vi "Ver 1.1.vi"() -> ()   [LabVIEW 2015]
uses:
  Program Files (x86)/National Instruments/LabVIEW 2016/instr.lib/Keithley 2000/Keithley 2000.lvlib
  Program Files (x86)/National Instruments/LabVIEW 2016/instr.lib/Keithley622xLV2009_0/Keithley 622x LV 2009/Keithley 622x.lvlib
  Program Files (x86)/National Instruments/LabVIEW 2016/instr.lib/Keithley622xLV2009_0/Keithley 622x LV 2009/Utility/Typedefs/KE622x -- Instrument Type.ctl
  Program Files (x86)/National Instruments/LabVIEW 2016/instr.lib/Keithley622xLV2009_0/Keithley 622x LV 2009/Configure/Source/Typedefs/KE622x -- Current Level.ctl
  Program Files (x86)/National Instruments/LabVIEW 2016/instr.lib/Keithley622xLV2009_0/Keithley 622x LV 2009/Configure/Source/Typedefs/KE622x -- Voltage Limit.ctl
  Program Files (x86)/National Instruments/LabVIEW 2016/instr.lib/Keithley 2000/Public/Configure/Configure DC Volts.vi
  Program Files (x86)/National Instruments/LabVIEW 2016/instr.lib/Keithley622xLV2009_0/Keithley 622x LV 2009/Typedefs/KE622x -- On Off Control.ctl
  Program Files (x86)/National Instruments/LabVIEW 2016/instr.lib/Keithley622xLV2009_0/Keithley 622x LV 2009/Configure/Source/Typedefs/KE622x -- Current Range.ctl
  Program Files (x86)/National Instruments/LabVIEW 2016/instr.lib/Keithley622xLV2009_0/Keithley 622x LV 2009/Configure/Source/Typedefs/KE622x -- Current Ranges.ctl
panel:
  out "Error Code":string
  in  "File name":string
  in  "Comments":string
  in  "Root Path":path=path "C:/"
  out "file":refnum<file>
  in  "Custom Range (0 V) 2":dbl format="%#_6p"
  in  "Auto\nRange 2":bool
  out "2000":refnum<visa-resource-name>
  out "6221":refnum<visa-resource-name>
  in  "Floating-point file recording":bool
  in  "Step  (A)":dbl=5e-05 format="%#_3p"
  in  "Stop\ncurrent (A)":dbl=0.002 format="%#_6p"
  in  "Start \ncurrent (A)":dbl=0.001 format="%#_6p"
  out "?":string
  out "?":string
  in  "Change Volt Ampers":bool
  in  "Check For SCPI Errors? (T)":bool=TRUE
  out "Interlock Tripped?":bool
  out "Compliance?":bool
  in  "Turn Off Output \nIf Compliance?":bool=TRUE
  in  "Turning ON/OFF\ncurrent output":T1=enum."On"
  out "?":cluster{dbl[], dbl[]}[](graph)
  in  "Range Selection":T2={"Auto Range?"=TRUE, "Man / Selected\nRange"=enum."2nA"}
  in  "Voltage Limit (V) 3":T4=10.0 min=0.1 max=105.0 step=0.01 format="%.2p"
  in  "Interval (s)":dbl=1.0 min=1.0
  out "?":cluster{T4[], T4[]}(graph)
  # "FILE CONFIGURATION"
  # "START, STOP, STEP, CONFIGURATION"
  # "KEITHLEY 6221 CONFIGURATION (ADMIN ONLY)"
  # "IF ON"
  # "I don't know what the hell it is,\njust don't touch it"
  # "Compliance = Limiting output voltage\nThis switch determines if we want to switch \noff the current output if wee exceed compliance"
  # "There is a safe switch at \nthe back of the instrument \nThis indicator shows if it is on"
  # "You have hit a damn jackpot \nby exceeding the limited voltage\nCongrats"
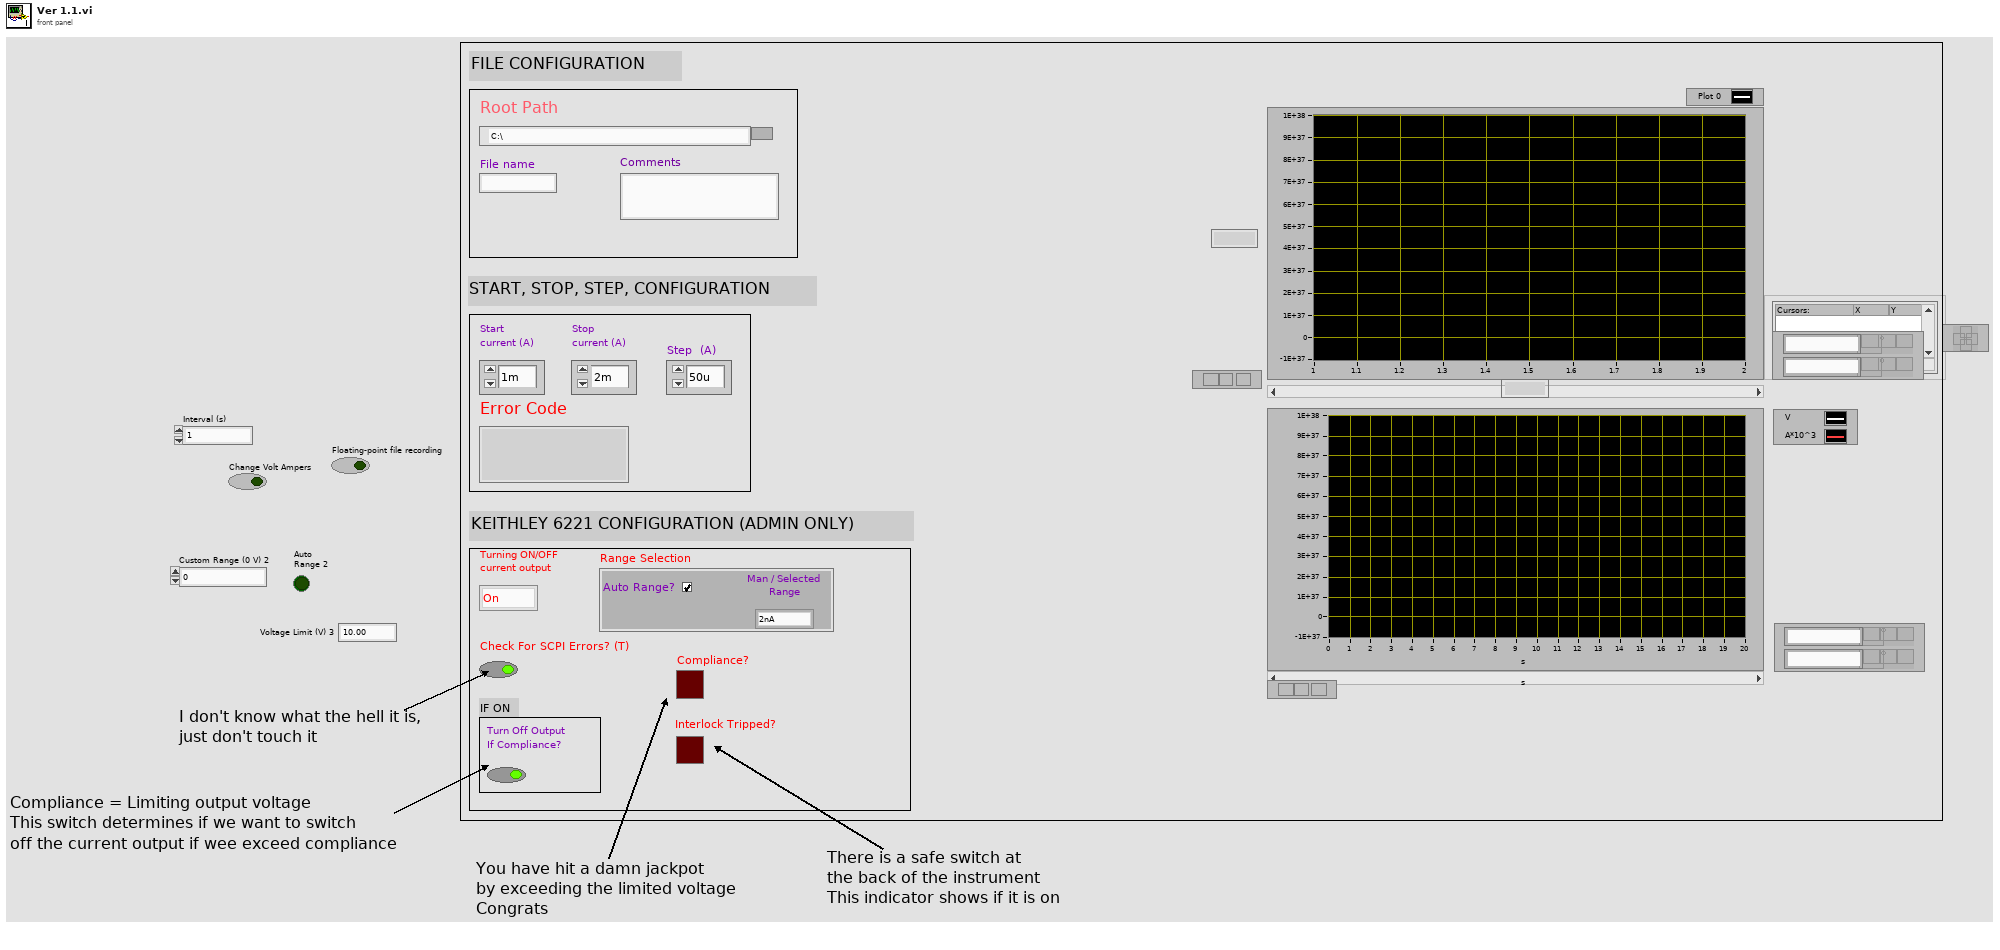
[diagram p1: front panel]
types:
  T1 = typedef "Keithley 622x.lvlib/KE622x -- On Off Control.ctl" = enum16{"Off", "On"}
  T2 = typedef "Keithley 622x.lvlib/KE622x -- Current Range.ctl" = cluster{"Auto Range?":bool, "Man / Selected\nRange":T3}
  T3 = typedef "Keithley 622x.lvlib/KE622x -- Current Ranges.ctl" = enum16{"2nA", "20nA", "200nA", "2uA", "20uA", "200uA", "2mA", "20mA", "100mA"}
  T4 = typedef "Keithley 622x.lvlib/KE622x -- Voltage Limit.ctl" = dbl
  T5 = enum16{"open", "replace", "create", "open or create", "replace or create", "replace or create with confirmation"}
  T6 = typedef "Keithley 622x.lvlib/KE622x -- Instrument Type.ctl" = enum16{"KE6220", "KE6221"}
  T7 = typedef "Keithley 622x.lvlib/KE622x -- Current Level.ctl" = dbl
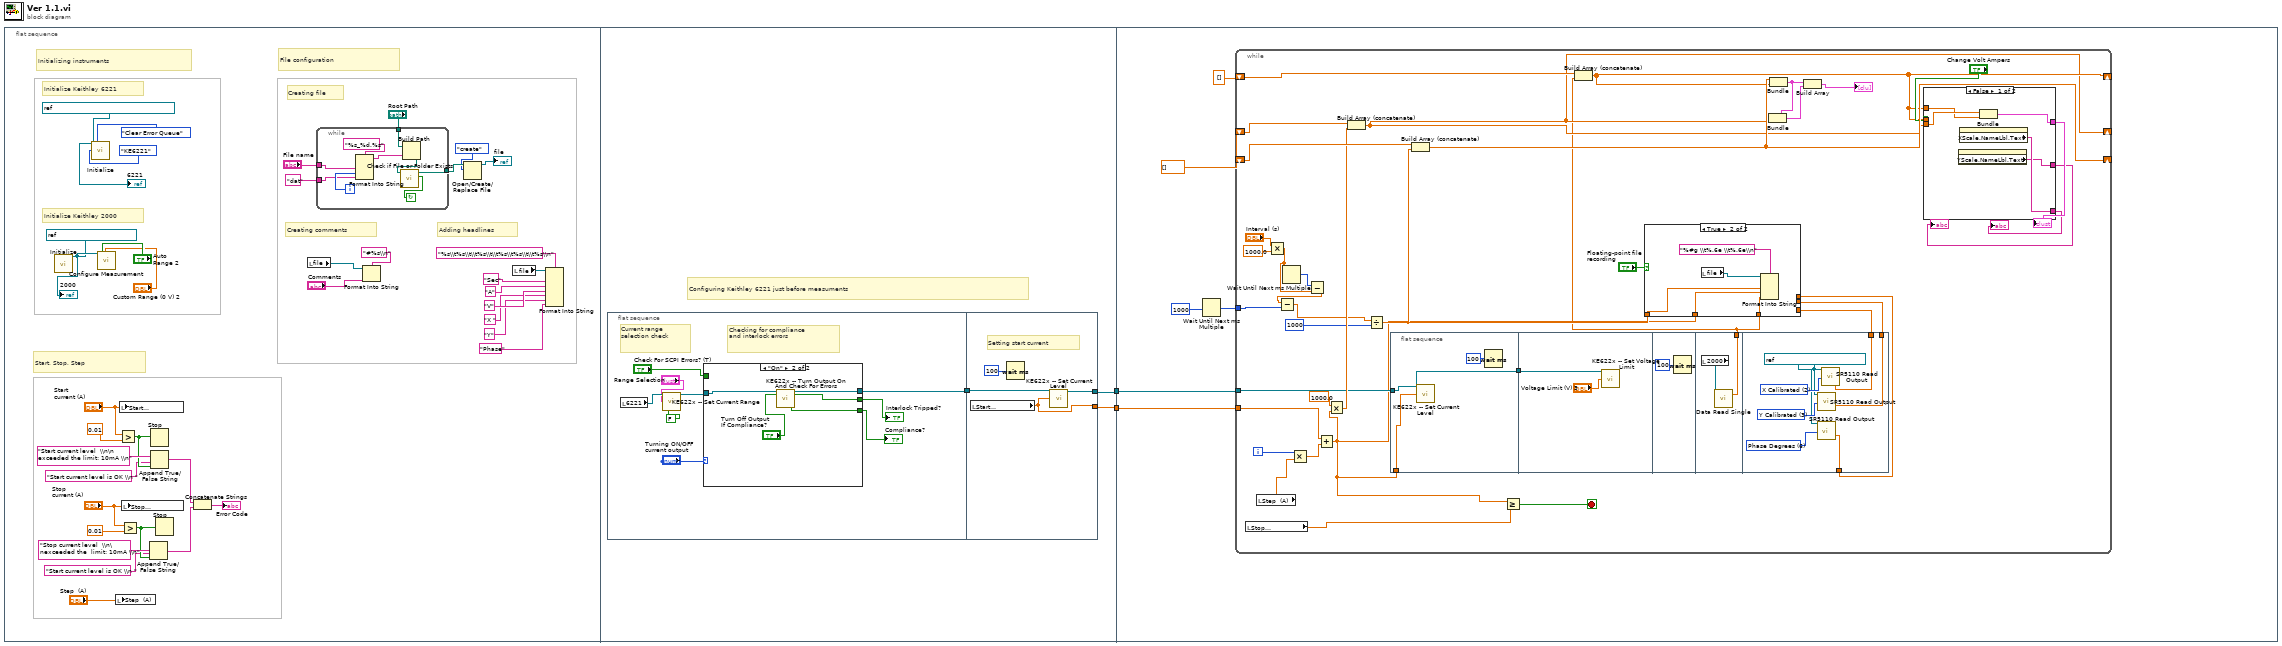
[diagram p0: block diagram]
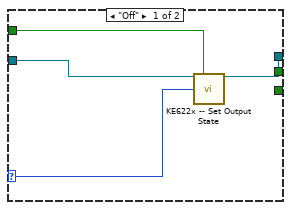
[diagram p2: hidden frame]
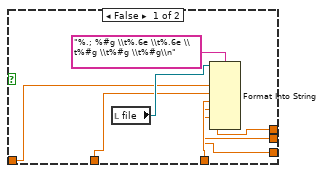
[diagram p3: hidden frame]
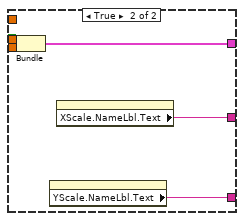
[diagram p4: hidden frame]
diagram:
  n1 = flat-sequence {
    tunnel: [w53] -> w2
    tunnel: [w52] -> w1
    tunnel: w2 -> [w76]
    tunnel: w1 -> [w77]
    frame #0 {
      # "Start, Stop, Step"
      # "Adding headlines"
      # "Creating file"
      # "Initializing instruments"
      # "Creating comments"
      # "File configuration"
      # "Initialize Keithley 2000"
      # "Initialize Keithley 6221"
      n2 = call "Initialize.vi"("VISA resource name"=refnum<visa-resource-name> "KEITHLEY_MULTIMETER") -> ("VISA resource name out"=w37:refnum<visa-resource-name>)  [unwired: 17 in, 1 out]
      "2000" <- w37
      n3 = call "Initialize.vi"("VISA resource name"=refnum<visa-resource-name> "KEITHLEY_DC_AC_CURRENT_SOURCE", "Error Queue Option"=enum16{"Clear Error Queue", "Error Query"}."Clear Error Queue", "Instrument Type"=KE622x_--_Instrument_Type."KE6221") -> ("VISA resource name out"=→"6221":refnum<visa-resource-name>)  [unwired: 11 in, 1 out]
      n4 = call-poly "Configure Measurement.vi"("VISA resource name"=w37, "Auto Range? (T: Auto)"="Auto\nRange 2", "Custom Range (0 V)"="Custom Range (0 V) 2") -> ()  [unwired: 15 in, 2 out]
      n5 = local write "Step  (A)"("Step  (A)") -> ()
      n6 = local write "Start \ncurrent (A)"("Start \ncurrent (A)") -> ()
      n7 = Greater?(x="Start \ncurrent (A)", y=T4 0.01) -> (0:w10:bool)
      n8 = Greater?(x="Stop\ncurrent (A)", y=T4 0.01) -> (0:w8:bool)
      n9 = local write "Stop\ncurrent (A)"("Stop\ncurrent (A)") -> ()
      n10 = Append True/False String(1:w8, 2:"Start current level is OK \\n " ("false string"), 3:"Stop current level  \\n\nexceeded the  limit: 10mA \\n" ("String")) -> (0:w4:string)  [unwired: 1 in]
      n11 = Stop(stop? (T)=w10) -> ()
      n12 = Append True/False String(1:w10, 2:"Start current level is OK \\n " ("false string"), 3:"Start current level  \\n\n exceeded the limit: 10mA \\n" ("String")) -> (0:w5:string)  [unwired: 1 in]
      n13 = Stop(stop? (T)=w8) -> ()
      n14 = Concatenate Strings(w5, w4) -> (→"Error Code":string)
      n15 = local read "file"() -> (w21:refnum<file>)
      n16 = while {
        tunnel: "dat" ("format string") -> [w48]
        tunnel: "File name" -> [w47]
        tunnel: "Root Path" -> [w45]
        tunnel: [w43] -> w31
        i -> [w49]
        stop <- w42 continue-if-true
        n17 = Format Into String(format string="%s_%d.%s", w47, w49, w48) -> (resulting string=w46:string)  [unwired: 2 in, 1 out]
        n18 = Build Path(base path=w45, name or relative path=w46) -> (appended path=w44:path)
        n19 = call <vilib>:"Check if File or Folder Exists.vi"("path"=w44) -> ("file or folder exists?"=w42:bool, "dup path"=w43:path)  [unwired: 8 in, 1 out]
      }
      n20 = Format Into String(format string="#%s\\n", initial string=w21, "Comments") -> ()  [unwired: 1 in, 2 out]
      n21 = Open/Create/Replace File(file path (use dialog)=w31, operation (0:open)=T5."create") -> (refnum out=→"file":refnum<file>)  [unwired: 4 in, 2 out]
      n22 = local read "file"() -> (w18:refnum<file>)
      n23 = Format Into String(format string="%s\\t%s\\t\\t%s\\t\\t%s\\t%s\\t\\t%s\\n", initial string=w18, "Sec" ("input 1"), "A" ("input 2"), "V" ("input 3"), "X " ("input 3"), "Y" ("input 3"), "Phase" ("input 3")) -> ()  [unwired: 1 in, 2 out]
    }
    frame #1 {
      # "Configuring Keithley 6221 just before measuments"
      n24 = flat-sequence {
        tunnel: [w54] -> w51
        tunnel: [w72] -> w53
        tunnel: [w74] -> w52
        tunnel: w51 -> [w73]
        frame #0 {
          # "Current range \nselection check"
          # "Checking for compliance\nand interlock errors"
          n25 = local read "6221"() -> (w57:refnum<visa-resource-name>)
          n26 = call "KE622x -- Set Current Range.vi"("Resource In"=w57, "Current Range In"="Range Selection", "Read Back Set Values? (T)"=FALSE) -> ("Resource Out (dupl)"=w62:refnum<visa-resource-name>)  [unwired: 10 in, 2 out]
          n27 = case shown="\"On\"" "Turning ON/OFF\ncurrent output" {
            selector: "Turning ON/OFF\ncurrent output" -> [w66 _]
            tunnel: [_ w70] -> w60
            tunnel: [_ w69] -> w61
            tunnel: "Check For SCPI Errors? (T)" -> [w65 _]
            tunnel: w62 -> [w63 w68]
            tunnel: [w64 w67] -> w54
            frame "Off" {
              n28 = call "KE622x -- Set Output State.vi"("Resource In"=w63, "Check For SCPI Errors? (T)"=w65, "Output State"=w66) -> ("Resource Out (dupl)"=w64:refnum<visa-resource-name>)  [unwired: 11 in, 1 out]
            }
            frame "On" {
              n29 = call "KE622x -- Turn Output On And Check For Errors.vi"("Resource In"=w68, "Turn Off Output If Compliance?"="Turn Off Output \nIf Compliance?") -> ("Resource Out (dupl)"=w67:refnum<visa-resource-name>, "Interlock Tripped?"=w70:bool, "Compliance?"=w69:bool)  [unwired: 10 in, 1 out]
            }
          }
          "Interlock Tripped?" <- w60
          "Compliance?" <- w61
        }
        frame #1 {
          # "Setting start current"
          n30 = local read "Start \ncurrent (A)"() -> (w72:dbl)
          n31 = Wait (ms)(milliseconds to wait=u32 100) -> ()  [unwired: 1 out]
          n32 = call "KE622x -- Set Current Level.vi"("Resource In"=w73, "Current Level (A) In"=w72) -> ("Resource Out (dupl)"=w74:refnum<visa-resource-name>)  [unwired: 11 in, 2 out]
        }
      }
    }
    frame #2 {
      n33 = Wait Until Next ms Multiple(millisecond multiple=u32 1000) -> (millisecond timer value=w78:u32)
      n34 = while {
        shift-right: [w110] -> _
        shift-left: dbl[] [] -> [w119]
        shift-right: [w115] -> _
        shift-left: _ -> [w117]
        shift-right: [w105] -> _
        shift-left: T7[] [] -> [w116]
        tunnel: w77 -> [w98]
        tunnel: w78 -> [w93]
        tunnel: w76 -> [w84]
        i -> [w107]
        stop <- w82 stop-if-true
        n35 = local read "Stop\ncurrent (A)"() -> (w83:dbl)
        n36 = local read "Step  (A)"() -> (w85:dbl)
        n37 = Multiply(x="Interval (s)", y=1000.0) -> (x*y=w94:dbl)
        n38 = Wait Until Next ms Multiple(millisecond multiple=w94) -> (millisecond timer value=w97:u32)
        n39 = Multiply(x=w107, y=w85) -> (x*y=w106:dbl)
        n40 = Subtract(x=w97, y=w94) -> (x-y=w92:dbl)
        n41 = Subtract(x=w92, y=w93) -> (x-y=w91:dbl)
        n42 = Add(x=w84, y=w106) -> (x+y=w95:dbl)
        n43 = Multiply(x=T4 1000.0, y=w95) -> (x*y=w104:T4)
        n44 = Build Array (concatenate)(w116, w104) -> (w105:T4[])
        n45 = Divide(x=w91, y=1000) -> (x/y=w101:dbl)
        n46 = flat-sequence {
          tunnel: w95 -> [w136]
          tunnel: w98 -> [w135]
          tunnel: [w134] -> w96
          tunnel: w96 -> [w137]
          tunnel: [w140] -> w88
          tunnel: [w148] -> w89
          tunnel: [w143] -> w87
          tunnel: [w142] -> w86
          frame #0 {
            n47 = call "KE622x -- Set Current Level.vi"("Resource In"=w135, "Current Level (A) In"=w136) -> ("Resource Out (dupl)"=w134:refnum<visa-resource-name>)  [unwired: 11 in, 2 out]
            n48 = Wait (ms)(milliseconds to wait=u32 100) -> ()  [unwired: 1 out]
          }
          frame #1 {
            n49 = call "KE622x -- Set Voltage Limit.vi"("Resource In"=w137, "Voltage Limit (V)"="Voltage Limit (V) 3") -> ()  [unwired: 12 in, 2 out]
          }
          frame #2 {
            n50 = Wait (ms)(milliseconds to wait=u32 100) -> ()  [unwired: 1 out]
          }
          frame #3 {
            n51 = local read "2000"() -> (w141:refnum<visa-resource-name>)
            n52 = call "Data Read Single.vi"("VISA resource name"=w141) -> ("Measurement"=w140:dbl)  [unwired: 14 in, 4 out]
          }
          frame #4 {
            w145 = u16 6 items=["X %", "Y %", "X Calibrated", "Y Calibrated", "Mag %", "Mag Calibrated", "Phase Degrees", "Ratio", "ADC 1", "ADC 2", "ADC 3", "ADC 4 ", "Noise %", "Noise Calibrated", "Ref Frequency", "", ""] ("Display Type")
            w146 = u16 3 items=["X %", "Y %", "X Calibrated", "Y Calibrated", "Mag %", "Mag Calibrated", "Phase Degrees", "Ratio", "ADC 1", "ADC 2", "ADC 3", "ADC 4 ", "Noise %", "Noise Calibrated", "Ref Frequency", "", ""] ("Display Type")
            w147 = u16 2 items=["X %", "Y %", "X Calibrated", "Y Calibrated", "Mag %", "Mag Calibrated", "Phase Degrees", "Ratio", "ADC 1", "ADC 2", "ADC 3", "ADC 4 ", "Noise %", "Noise Calibrated", "Ref Frequency", "", ""] ("Display Type")
            w144 = refnum<visa-resource-name> "LOCK_IN_5110_PRINCETON" ("VISA session (for class)")
            n53 = call "SR5110 Read Output"("VISA session (for class)"=w144, "Display Type"=w145) -> ("Output (FP)"=w142:dbl)  [unwired: 9 in, 8 out]
            n54 = call "SR5110 Read Output"("VISA session (for class)"=w144, "Display Type"=w146) -> ("Output (FP)"=w143:dbl)  [unwired: 9 in, 8 out]
            n55 = call "SR5110 Read Output"("VISA session (for class)"=w144, "Display Type"=w147) -> ("Display"=w148:dbl)  [unwired: 9 in, 8 out]
          }
        }
        n56 = Build Array (concatenate)(w117, w101) -> (w115:dbl[])
        n57 = Greater Or Equal?(x=w95, y=w83) -> (x >= y?=w82:bool)
        n58 = Build Array (concatenate)(w119, w88) -> (w110:dbl[])
        n59 = case shown="True" "Floating-point file recording" {
          tunnel: w101 -> [w123 w130]
          tunnel: w88 -> [w125 w129]
          tunnel: w95 -> [w124 w128]
          tunnel: w89 -> [w122 _]
          tunnel: w87 -> [w121 _]
          tunnel: w86 -> [w120 _]
          frame False {
            n60 = local read "file"() -> (w126:refnum<file>)
            n61 = Format Into String(format string="%.; %#g \\t%.6e \\t%.6e \\t%#g \\t%#g \\t%#g\\n", initial string=w126, w123, w124, w125, w122, w121, w120) -> ()  [unwired: 1 in, 2 out]
          }
          frame True {
            n62 = local read "file"() -> (w131:refnum<file>)
            n63 = Format Into String(format string="%#g \\t%.6e \\t%.6e\\n", initial string=w131, w130, w128, w129) -> ()  [unwired: 1 in, 2 out]
          }
        }
        n64 = Bundle(w115, w110) -> (w113:cluster{dbl[], dbl[]})  [unwired: 1 in]
        n65 = Bundle(cluster=w113, w105) -> (w114:cluster{dbl[], dbl[]})  [unwired: 1 in]
        n66 = Build Array(w113, w114) -> (→"?":cluster{dbl[], dbl[]}[])
        n67 = case shown="False" "Change Volt Ampers" {
          tunnel: [w153 w158] -> w118
          tunnel: w110 -> [_ w157]
          tunnel: w105 -> [w152 w156]
          tunnel: w110 -> [w151 _]
          tunnel: [w149 w155] -> w109
          tunnel: [w150 w154] -> w108
          frame False {
            n68 = property class="XYGraph (strict)"() -> ("YScale.NameLbl.Text"=w149:string)  [unwired: 2 in, 2 out]
            n69 = property class="XYGraph (strict)"() -> ("XScale.NameLbl.Text"=w150:string)  [unwired: 2 in, 2 out]
            n70 = Bundle(w152, w151) -> (w153:cluster{T4[], dbl[]})  [unwired: 1 in]
          }
          frame True {
            n71 = Bundle(w157, w156) -> (w158:cluster{dbl[], T4[]})  [unwired: 1 in]
            n72 = property class="XYGraph (strict)"() -> ("YScale.NameLbl.Text"=w154:string)  [unwired: 2 in, 2 out]
            n73 = property class="XYGraph (strict)"() -> ("XScale.NameLbl.Text"=w155:string)  [unwired: 2 in, 2 out]
          }
        }
        "?" <- w118
        "?" <- w109
        "?" <- w108
      }
    }
  }
